vi "startAutomatedTest.vi"(8 "error in (no error)":errorcluster, 10 "model":refnum<class "Model.lvclass">, 11 "InteractiveMotionState in":refnum<class "InteractiveMotionState.lvclass">) -> (0 "error out":errorcluster, 2 "model 2":refnum<class "Model.lvclass">, 3 "InteractiveMotionState out":refnum<class "InteractiveMotionState.lvclass">)   [LabVIEW 2015, in "InteractiveMotionState.lvclass"]
uses:
  InteractiveMotionState.lvclass
  Model/Model/Model.lvclass
  Typedefs/StateSelector.ctl
  Typedefs/M1M3SSSTypedefs.lvlib
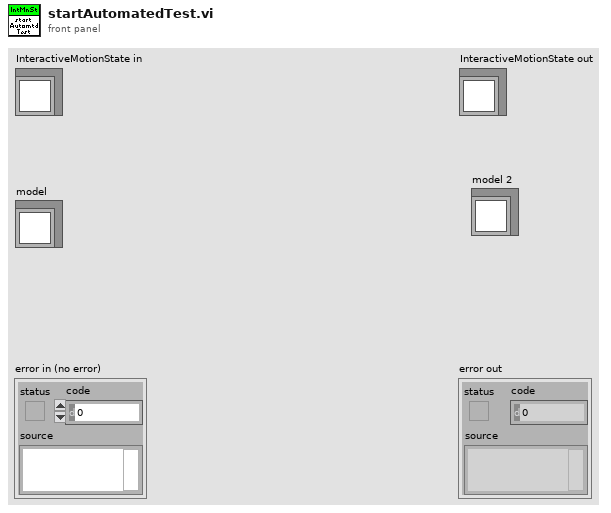
[diagram p1: front panel]
types:
  T1 = typedef "M1M3SSSTypedefs.lvlib/StateSelector.ctl" = enum16{"FaultState", "OffState", "RampingUpPressurePState", "RampingUpPressureSTState", "StandbyState", "StoppedState", "WaitingForSettledPState", "WaitingForSettledSTState"}
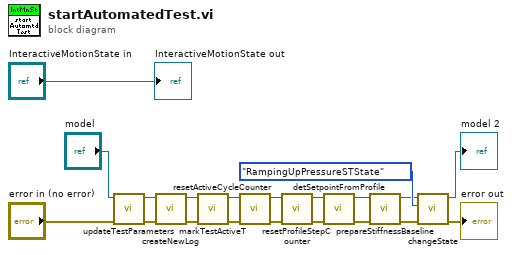
[diagram p0: block diagram]
diagram:
  n1 = call "updateTestParameters.vi"("error in (no error)"="error in (no error)", "Model in"="model") -> ("error out"=w9:errorcluster, "Model out"=w11:refnum<class "Model.lvclass">)  [unwired: 8 in]
  n2 = call "createNewLog.vi"("error in (no error)"=w9, "Model in"=w11) -> ("error out"=w14:errorcluster, "Model out"=w16:refnum<class "Model.lvclass">)  [unwired: 8 in]
  n3 = call "markTestActiveT.vi"("error in (no error)"=w14, "Model in"=w16) -> ("error out"=w13:errorcluster, "Model out"=w15:refnum<class "Model.lvclass">)  [unwired: 8 in]
  n4 = call "resetActiveCycleCounter.vi"("error in (no error)"=w13, "Model in"=w15) -> ("error out"=w1:errorcluster, "Model out"=w2:refnum<class "Model.lvclass">)  [unwired: 8 in]
  n5 = call "resetProfileStepCounter.vi"("error in (no error)"=w1, "Model in"=w2) -> ("error out"=w7:errorcluster, "Model out"=w8:refnum<class "Model.lvclass">)  [unwired: 8 in]
  n6 = call "detSetpointFromProfile.vi"("error in (no error)"=w7, "Model in"=w8) -> ("error out"=w4:errorcluster, "Model out"=w6:refnum<class "Model.lvclass">)  [unwired: 8 in]
  n7 = call "prepareStiffnessBaseline.vi"("error in (no error)"=w4, "Model in"=w6) -> ("error out"=w3:errorcluster, "Model out"=w5:refnum<class "Model.lvclass">)  [unwired: 8 in]
  n8 = call "changeState.vi"("error in (no error)"=w3, "State:"=StateSelector."RampingUpPressureSTState", "Model in"=w5) -> ("error out"=→"error out":errorcluster, "Model out"=→"model 2":refnum<class "Model.lvclass">)  [unwired: 7 in]
  "InteractiveMotionState out" <- "InteractiveMotionState in"
